vi "Configure FlexRay Sessions and Start.vi"(8 "error in (no error)":errorcluster, 10 "Device Reference in":T1 format="%.0x", 11 "cluster in":T5 {"ctrl_stat"."ctrl_state" format="%.0x"; "FRConfig"."Output Refs" format="%.0x"; "FRConfig"."Input Refs" format="%.0x"; "FRConfig"."EventFrames list"."Channel Data Ref" format="%.0x"}) -> (0 "error out":errorcluster, 3 "cluster out":T5 {"ctrl_stat"."ctrl_state" format="%.0x"; "FRConfig"."Output Refs" format="%.0x"; "FRConfig"."Input Refs" format="%.0x"; "FRConfig"."EventFrames list"."Channel Data Ref" format="%.0x"})   [LabVIEW 2020, in "FlexRay Custom Device Engine.lvlib"]
uses:
  FlexRay Custom Device Engine.lvlib
  <vilib>/NI VeriStand/Custom Device API/Custom Device Item Ref.ctl
  <vilib>/NI VeriStand/Custom Device API/Data Reference.ctl
  Shared/FREventInfo.ctl
  Shared/InterfaceState.ctl
  Shared/FRConfig.ctl
  Shared/FRInterface.ctl
  <vilib>/xnet/xnet.llb/XNET Control Scope.ctl
  Shared/Constants.vi
  <vilib>/NI VeriStand/Custom Device API/Get Item Property (Variant).vi
  <vilib>/xnet/xnet.llb/XNET Create Session (Signal Output Single-point).vi
  <vilib>/xnet/xnet.llb/XNET Create Session (Signal Input Single-point).vi
  <vilib>/NI VeriStand/Custom Device API/Custom Device API.lvlib
  Shared/FlexRay Custom Device Shared.lvlib
  <resource>/objmgr/xnet.rc
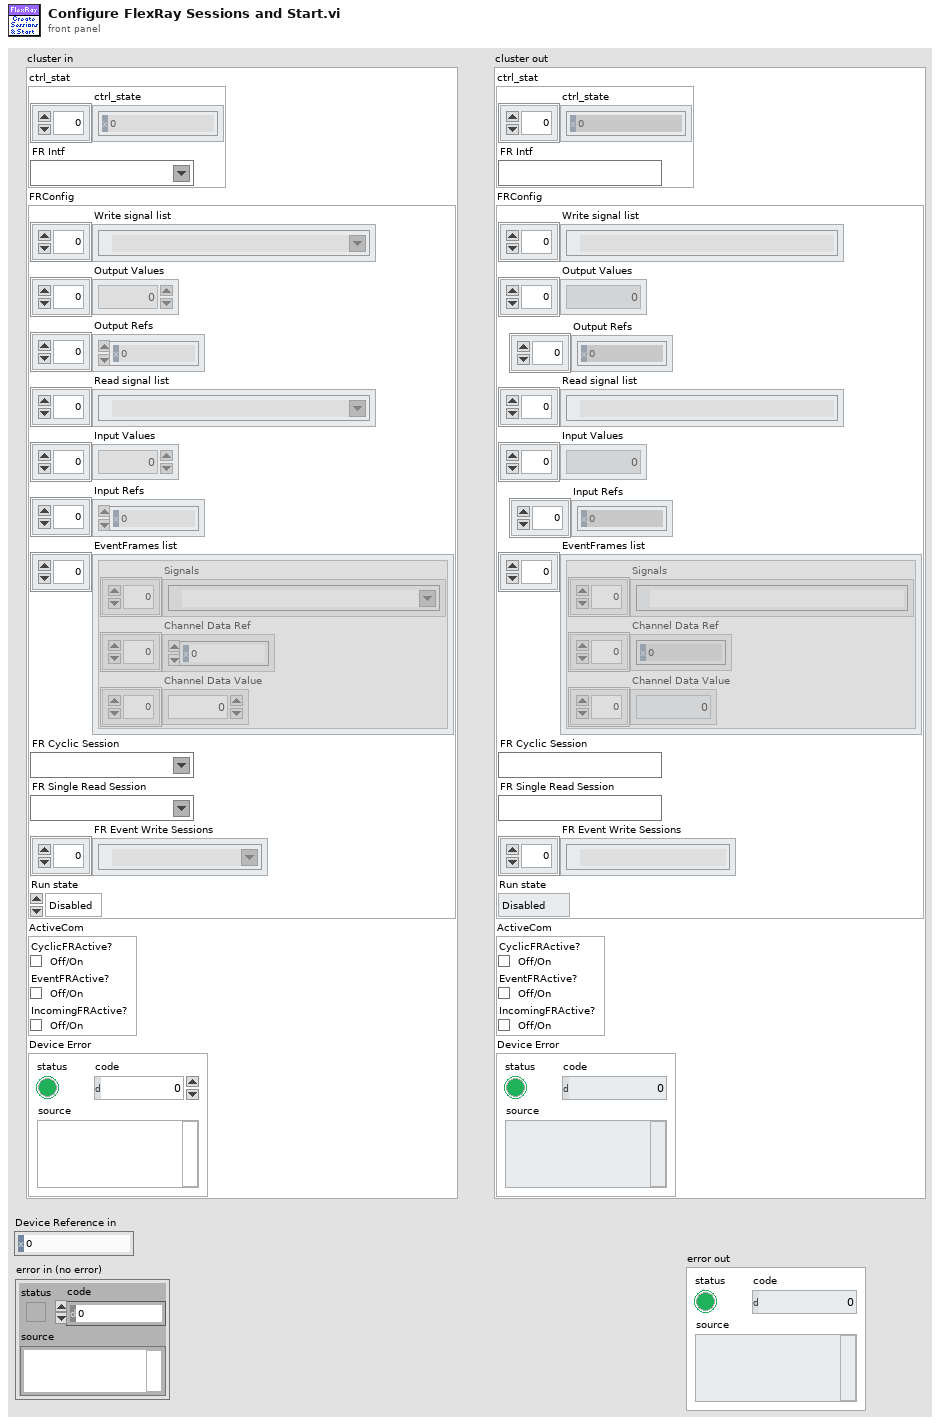
[diagram p1: front panel]
types:
  T1 = typedef "Custom Device API.lvlib/Custom Device Item Ref.ctl" = u64
  T2 = typedef "Custom Device API.lvlib/Data Reference.ctl" = i32
  T3 = typedef "FlexRay Custom Device Shared.lvlib/FREventInfo.ctl" = cluster{"Signals":refnum<k21>[], "Channel Data Ref":T2[], "Channel Data Value":dbl[]}
  T4 = typedef "FlexRay Custom Device Engine.lvlib/InterfaceState.ctl" = enum16{"Disabled", "Enabled", "Init"}
  T5 = cluster{"ctrl_stat":cluster{"ctrl_state":T1[], "FR Intf":refnum<k21>}, "FRConfig":cluster{"Write signal list":refnum<k21>[], "Output Values":dbl[], "Output Refs":T2[], "Read signal list":refnum<k21>[], "Input Values":dbl[], "Input Refs":T2[], "EventFrames list":T3[], "FR Cyclic Session":refnum<k21>, "FR Single Read Session":refnum<k21>, "FR Event Write Sessions":refnum<k21>[], "Run state":T4}, "ActiveCom":cluster{"CyclicFRActive?":bool, "EventFRActive?":bool, "IncomingFRActive?":bool}, "Device Error":errorcluster}
  T6 = typedef "FlexRay Custom Device Shared.lvlib/FRConfig.ctl" = cluster{"FlexRay Interface":T7, "XNET Database":refnum<k21>, "XNET Cluster":refnum<k21>, "ColdStart ID":u32, "Termination":bool}
  T7 = typedef "FlexRay Custom Device Shared.lvlib/FRInterface.ctl" = u16
  T8 = typedef "XNET Control Scope.ctl" = u32
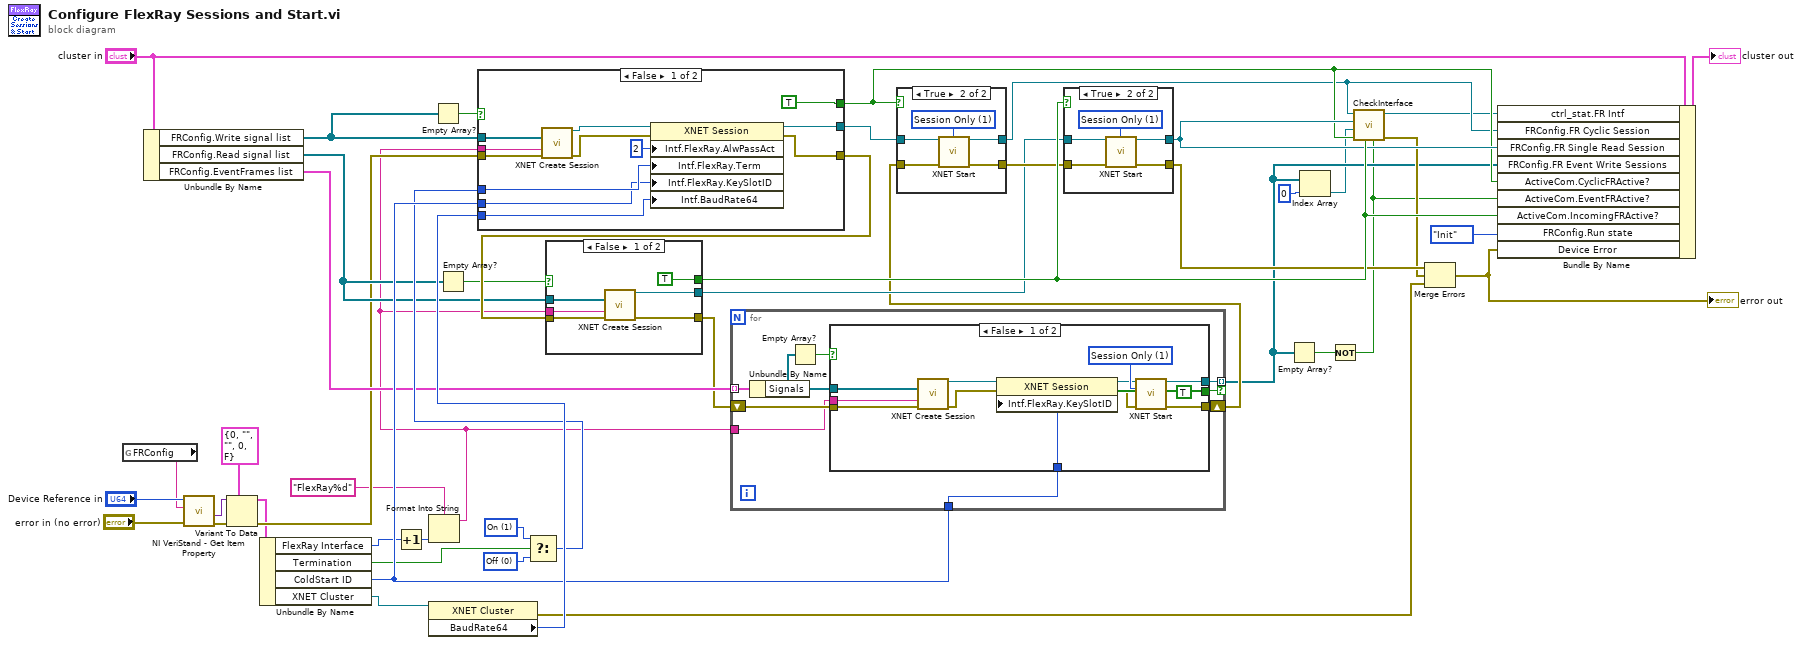
[diagram p0: block diagram]
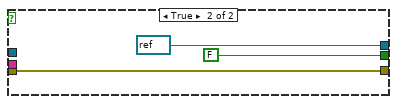
[diagram p4: hidden frame]
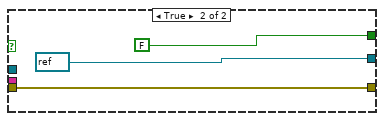
[diagram p5: hidden frame]
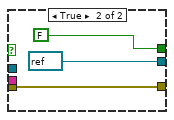
[diagram p6: hidden frame]
diagram:
  w17 = u32 1 items=["Off", "On"] ("Interface:FlexRay:Termination")
  w18 = u32 0 items=["Off", "On"] ("Interface:FlexRay:Termination")
  n1 = global read "Constants.vi" "FRConfig"() -> (w5:string)
  n2 = Unbundle By Name("cluster in") -> ("FRConfig.Write signal list"=w25:refnum<k21>[], "FRConfig.Read signal list"=w24:refnum<k21>[], "FRConfig.EventFrames list"=w26:T3[])
  n3 = call-poly <vilib>:"NI VeriStand - Get Item Property.vi"("error in (no error)"="error in (no error)", "Property Name"=w5, "Item Ref in"="Device Reference in") -> ("error out"=w6:errorcluster, "Value"=w7:variant)  [unwired: 5 in, 2 out]
  n4 = Variant To Data(error in=w6, type=T6 {"FlexRay Interface"=0, "XNET Database"="", "XNET Cluster"="", "ColdStart ID"=0, "Termination"=FALSE} ("FRConfig"), Variant=w7) -> (data=w9:T6, error out=w15:errorcluster)
  n5 = Unbundle By Name(w9) -> ("FlexRay Interface"=w10:T7, "Termination"=w16:bool, "ColdStart ID"=w36:u32, "XNET Cluster"=w21:refnum<k21>)
  n6 = Increment(x=w10) -> (x+1=w11:T7)
  n7 = Format Into String(format string="FlexRay%d", w11) -> (resulting string=w14:string)  [unwired: 2 in, 1 out]
  n8 = property class="XNET Cluster"(reference=w21) -> (error out=w28:errorcluster, "BaudRate64"=w37:u64)  [unwired: 1 in, 1 out]
  n9 = Empty Array?(array=w25) -> (empty?=w19:bool)
  n10 = Empty Array?(array=w24) -> (empty?=w20:bool)
  n11 = Select(t=w17, s=w16, f=w18) -> (s? t:f=w35:u32)
  n12 = case shown="False" w19 {
    tunnel: [w48 refnum<k21> refnum ("session out")] -> w39
    tunnel: w25 -> [w59 _]
    tunnel: [w49 w62] -> w40
    tunnel: w14 -> [w58 _]
    tunnel: w15 -> [w57 w62]
    tunnel: [TRUE FALSE] -> w41
    tunnel: w35 -> [w53 _]
    tunnel: w36 -> [w52 _]
    tunnel: w37 -> [w50 _]
    frame False {
      n13 = call-poly <vilib>:"XNET Create Session.vi"("signal list"=w59, "interface"=w58, "error in (no error)"=w57) -> ("session out"=w55:refnum<k21>, "error out"=w54:errorcluster)  [unwired: 11 in]
      n14 = property class="XNET Session"(reference=w55, error in=w54, "Intf.FlexRay.AlwPassAct"=u32 2 ("Interface:FlexRay:Allow Passive to Active"), "Intf.FlexRay.Term"=w53, "Intf.FlexRay.KeySlotID"=w52, "Intf.BaudRate64"=w50) -> (reference out=w48:refnum<k21>, error out=w49:errorcluster)
    }
    frame True {
    }
  }
  n15 = case shown="False" w20 {
    tunnel: w24 -> [w68 _]
    tunnel: w40 -> [w67 w70]
    tunnel: [w64 refnum<k21> refnum ("session out")] -> w43
    tunnel: [w63 w70] -> w4
    tunnel: w14 -> [w66 _]
    tunnel: [TRUE FALSE] -> w47
    frame False {
      n16 = call-poly <vilib>:"XNET Create Session.vi"("signal list"=w68, "interface"=w66, "error in (no error)"=w67) -> ("session out"=w64:refnum<k21>, "error out"=w63:errorcluster)  [unwired: 11 in]
    }
    frame True {
    }
  }
  n17 = for {
    tunnel: w14 -> [w78]
    tunnel: [w73] -> w32 mode=indexing if=w74
    tunnel: w26 -> [w77] mode=indexing
    shift-right: [w79] -> w42
    shift-left: w4 -> [w80]
    tunnel: w36 -> [w72]
    n18 = Unbundle By Name(w77) -> ("Signals"=w76:refnum<k21>[])
    n19 = Empty Array?(array=w76) -> (empty?=w75:bool)
    n20 = case shown="False" w75 {
      tunnel: w80 -> [w92 w95]
      tunnel: [w89 w95] -> w79
      tunnel: [w90 refnum<k21> refnum ("session out")] -> w73
      tunnel: w78 -> [w91 _]
      tunnel: w76 -> [w86 _]
      tunnel: [TRUE FALSE] -> w74
      tunnel: w72 -> [w82 _]
      frame False {
        w88 = T8 1 items=["Normal", "Session Only", "Interface Only", "Session Only Blocking"] ("scope (normal)")
        n21 = call-poly <vilib>:"XNET Create Session.vi"("signal list"=w86, "interface"=w91, "error in (no error)"=w92) -> ("session out"=w85:refnum<k21>, "error out"=w81:errorcluster)  [unwired: 11 in]
        n22 = property class="XNET Session"(reference=w85, error in=w81, "Intf.FlexRay.KeySlotID"=w82) -> (reference out=w84:refnum<k21>, error out=w83:errorcluster)
        n23 = call <vilib>:"XNET Start.vi"("session in"=w84, "scope (normal)"=w88, "error in (no error)"=w83) -> ("session out"=w90:refnum<k21>, "error out"=w89:errorcluster)  [unwired: 11 in]
      }
      frame True {
      }
    }
  }
  n24 = case shown="True" w41 {
    tunnel: [w97 w101] -> w38
    tunnel: w39 -> [w97 w100]
    tunnel: w42 -> [w96 w99]
    tunnel: [w96 w98] -> w45
    frame False {
    }
    frame True {
      w102 = T8 1 items=["Normal", "Session Only", "Interface Only", "Session Only Blocking"] ("scope (normal)")
      n25 = call <vilib>:"XNET Start.vi"("session in"=w100, "scope (normal)"=w102, "error in (no error)"=w99) -> ("session out"=w101:refnum<k21>, "error out"=w98:errorcluster)  [unwired: 11 in]
    }
  }
  n26 = case shown="True" w47 {
    tunnel: [w104 w108] -> w44
    tunnel: w43 -> [w104 w107]
    tunnel: w45 -> [w103 w106]
    tunnel: [w103 w105] -> w46
    frame False {
    }
    frame True {
      w109 = T8 1 items=["Normal", "Session Only", "Interface Only", "Session Only Blocking"] ("scope (normal)")
      n27 = call <vilib>:"XNET Start.vi"("session in"=w107, "scope (normal)"=w109, "error in (no error)"=w106) -> ("session out"=w108:refnum<k21>, "error out"=w105:errorcluster)  [unwired: 11 in]
    }
  }
  n28 = Empty Array?(array=w32) -> (empty?=w27:bool)
  n29 = Index Array(array=w32, index=0) -> (element=w31:refnum<k21>)
  n30 = Not(x=w27) -> (.not. x?=w30:bool)
  n31 = call "CheckInterface.vi"("Ref 3 Active"=w30, "Ref 2 Active"=w47, "Ref 1 Active"=w41, "Ref 3"=w31, "Ref 2"=w44, "Ref 1"=w38) -> ("error out"=w34:errorcluster, "CtrlIntf"=w33:refnum<k21>)  [unwired: 4 in]
  n32 = Merge Errors(w46, w34, w28) -> (w23:errorcluster)
  "error out" <- w23
  n33 = Bundle By Name(cluster="cluster in", "ctrl_stat.FR Intf"=w33, "FRConfig.FR Cyclic Session"=w38, "FRConfig.FR Single Read Session"=w44, "FRConfig.FR Event Write Sessions"=w32, "ActiveCom.CyclicFRActive?"=w41, "ActiveCom.EventFRActive?"=w30, "ActiveCom.IncomingFRActive?"=w47, "FRConfig.Run state"=InterfaceState."Init", "Device Error"=w23) -> (→"cluster out":T5)
